vi "Main.vi"() -> ()   [LabVIEW 2014]
uses:
  <vilib>/vision/NI_Vision_Development_Module.lvlib
  <vilib>/vision/Measure.llb/Edge Polarity.ctl
  <vilib>/vision/Measure.llb/Edge Options.ctl
  <vilib>/vision/Measure.llb/Edge New.ctl
panel:
  out "Size factor":dbl
  in  "Tab Control":enum32{"MCF", "Kapilara"}(tab)
  in  "Nr punktu":i32
  in  "HIDE / SHOW":bool
  in  "Pole widzenia":dbl
  in  "Próg dopasowania okręgu":dbl=35.0
  in  "START":bool
  out "Mniejsza oś":dbl
  out "Większa oś":dbl
  out "Ekscentryczność":dbl
  out "Kołowość":dbl
  out "Przesunięcie [um]":dbl
  out "Parametry":string[][](table)
  in  "File path":path
  in  "START 2":bool
  in  "Pole widzenia":dbl
  in  "File path 2":path
  out "Średnica zewnętrzna [um]":i16
  out "Średnica wewnętrzna [um]":dbl format="%#_3g"
  in  "Options":T3={"Search  Direction"=1, "Edge Options"={"Edge Polarity"=2, "Kernel Size"=3, "Width"=3, "Minimum Edge Strength"=35.0, "Interpolation Type"=enum."Bilinear Fixed", "Data Processing Method"=enum."Average"}, "Show Search Area"=FALSE, "Show Search Lines"=FALSE, "Show Edges Found"=FALSE, "Show Result"=TRUE, "Search Area Color"=16711680, "Search Lines Color"=255, "Edge Locations Color"=16776960, "Result Color"=2162432, "Overlay Group Name"=""} {"Search  Direction" items=["Outside to Inside", "Inside to Outside"]; "Edge Options"."Edge Polarity" items=["All Edges", "Rising Edges", "Falling Edges"]; "Edge Options"."Minimum Edge Strength" format="%.2f"; "Edge Options"."Width" step=2; "Edge Options"."Kernel Size" step=2}
  in  "STOP":bool
  out "Array 3":cluster{"Edge Info":T4, "Boolean":bool}[](array[cluster]) {"Edge Info"."Distance (Real-World)" format="%.2f"; "Edge Info"."Location (Real-World)"."Y" format="%.2g"; "Edge Info"."Location (Real-World)"."X" format="%.2f"; "Edge Info"."Noise" format="%.2f"; "Edge Info"."Location (Pixel)"."Y" format="%.2g"; "Edge Info"."Location (Pixel)"."X" format="%.2f"; "Edge Info"."Strength" format="%.2f"; "Edge Info"."Distance (Pixel)" format="%.2f"}
  out "Displayed image":T5(plugin-control)
  out "Points array":cluster{"Edge Info":T4, "Boolean":bool}[](array[cluster]) {"Edge Info"."Distance (Real-World)" format="%.2f"; "Edge Info"."Location (Real-World)"."Y" format="%.2g"; "Edge Info"."Location (Real-World)"."X" format="%.2f"; "Edge Info"."Noise" format="%.2f"; "Edge Info"."Location (Pixel)"."Y" format="%.2g"; "Edge Info"."Location (Pixel)"."X" format="%.2f"; "Edge Info"."Strength" format="%.2f"; "Edge Info"."Distance (Pixel)" format="%.2f"}
  out "Original image":T5(plugin-control)
  # "Kliknięcie na zdjęciu spowoduje zaznaczenie \nnajbliższego punktu (widocznego lub ukrytego).\n\nNaciśnięcie przycisku POKAŻ / UKRYJ \nlub DOWOLNEGO PRZYCISKU NA KLAWIATURZE \nspowoduje pokazanie / ukrycie zaznaczonego punktu. \n\nDo obliczeń brane są tylko punkty widoczne na zdjęciu."
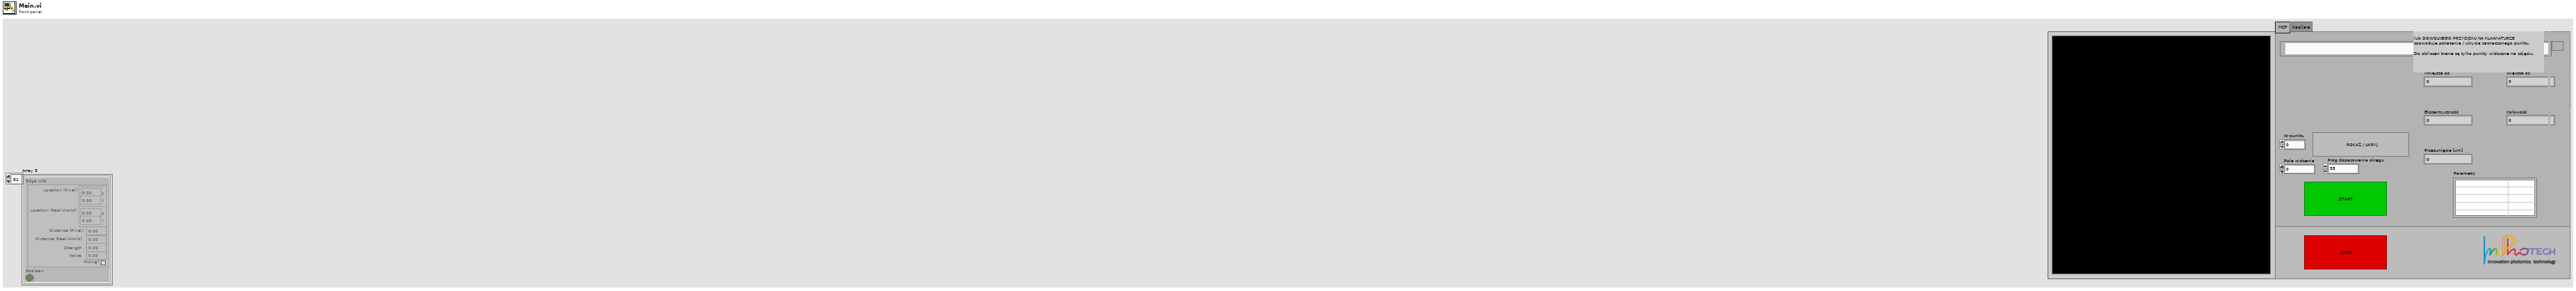
[diagram p1: front panel]
types:
  T1 = typedef "Edge Options.ctl" = cluster{"Edge Polarity":T2, "Kernel Size":u32, "Width":u32, "Minimum Edge Strength":sgl, "Interpolation Type":enum32{"Zero Order", "Bilinear", "Quadratic", "Cubic", "Bilinear Fixed"}, "Data Processing Method":enum32{"Average", "Median"}}
  T2 = typedef "Edge Polarity.ctl" = u32
  T3 = cluster{"Search  Direction":u32, "Edge Options":T1, "Show Search Area":bool, "Show Search Lines":bool, "Show Edges Found":bool, "Show Result":bool, "Search Area Color":u32, "Search Lines Color":u32, "Edge Locations Color":u32, "Result Color":u32, "Overlay Group Name":string}
  T4 = typedef "Edge New.ctl" = cluster{"Location (Pixel)":cluster{"X":sgl, "Y":sgl}, "Location (Real-World)":cluster{"X":sgl, "Y":sgl}, "Distance (Pixel)":dbl, "Distance (Real-World)":dbl, "Strength":dbl, "Noise":dbl, "Rising?":bool}
  T5 = typedef "IMAQ Image.ctl" = refnum<image>
  T6 = typedef "IMAQ Circle" = cluster{"Center X":i32, "Center Y":i32, "Inner Radius":i32, "Outer Radius":i32, "Start Angle":dbl, "End Angle":dbl}
  T7 = cluster{dbl, dbl, dbl, dbl, "Start Angle":dbl, "End Angle":dbl}
  T8 = typedef "ROI Descriptor" = cluster{"Global Rectangle":i32[], "Contours":cluster{"ID":enum32{"External", "Internal"}, "Type":u32, "Coordinates":i32[]}[]}
  T9 = cluster{"Center (Pixels)":cluster{"X":sgl, "Y":sgl}, "Radius (Pixels)":dbl, "Center (Real-World)":cluster{"X":sgl, "Y":sgl}, "Radius (Real-World)":dbl, "Roundness (Real-World)":dbl, "Average Strength":dbl, "Average SNR (dB)":dbl}
  T10 = cluster{"Center":cluster{"X":sgl, "Y":sgl}, "Major Axis":cluster{"Point 1":cluster{"X":sgl, "Y":sgl}, "Point 2":cluster{"X":sgl, "Y":sgl}}, "Minor Axis":cluster{"Point 1":cluster{"X":sgl, "Y":sgl}, "Point 2":cluster{"X":sgl, "Y":sgl}}}
  T11 = enum32{"Zero Order", "Bilinear", "Quadratic", "Cubic", "Bilinear Fixed"}
  T12 = cluster{"Edge Polarity":T2, "Kernel Size":u32, "Width":u32, "NewVal":dbl, "Interpolation Type":enum32{"Zero Order", "Bilinear", "Quadratic", "Cubic", "Bilinear Fixed"}, "Data Processing Method":enum32{"Average", "Median"}}
  T13 = cluster{"Search  Direction":u32, cluster{"Edge Polarity":T2, "Kernel Size":u32, "Width":u32, "NewVal":dbl, "Interpolation Type":enum32{"Zero Order", "Bilinear", "Quadratic", "Cubic", "Bilinear Fixed"}, "Data Processing Method":enum32{"Average", "Median"}}, "Show Search Area":bool, "Show Search Lines":bool, "Show Edges Found":bool, "Show Result":bool, "Search Area Color":u32, "Search Lines Color":u32, "Edge Locations Color":u32, "Result Color":u32, "Overlay Group Name":string}
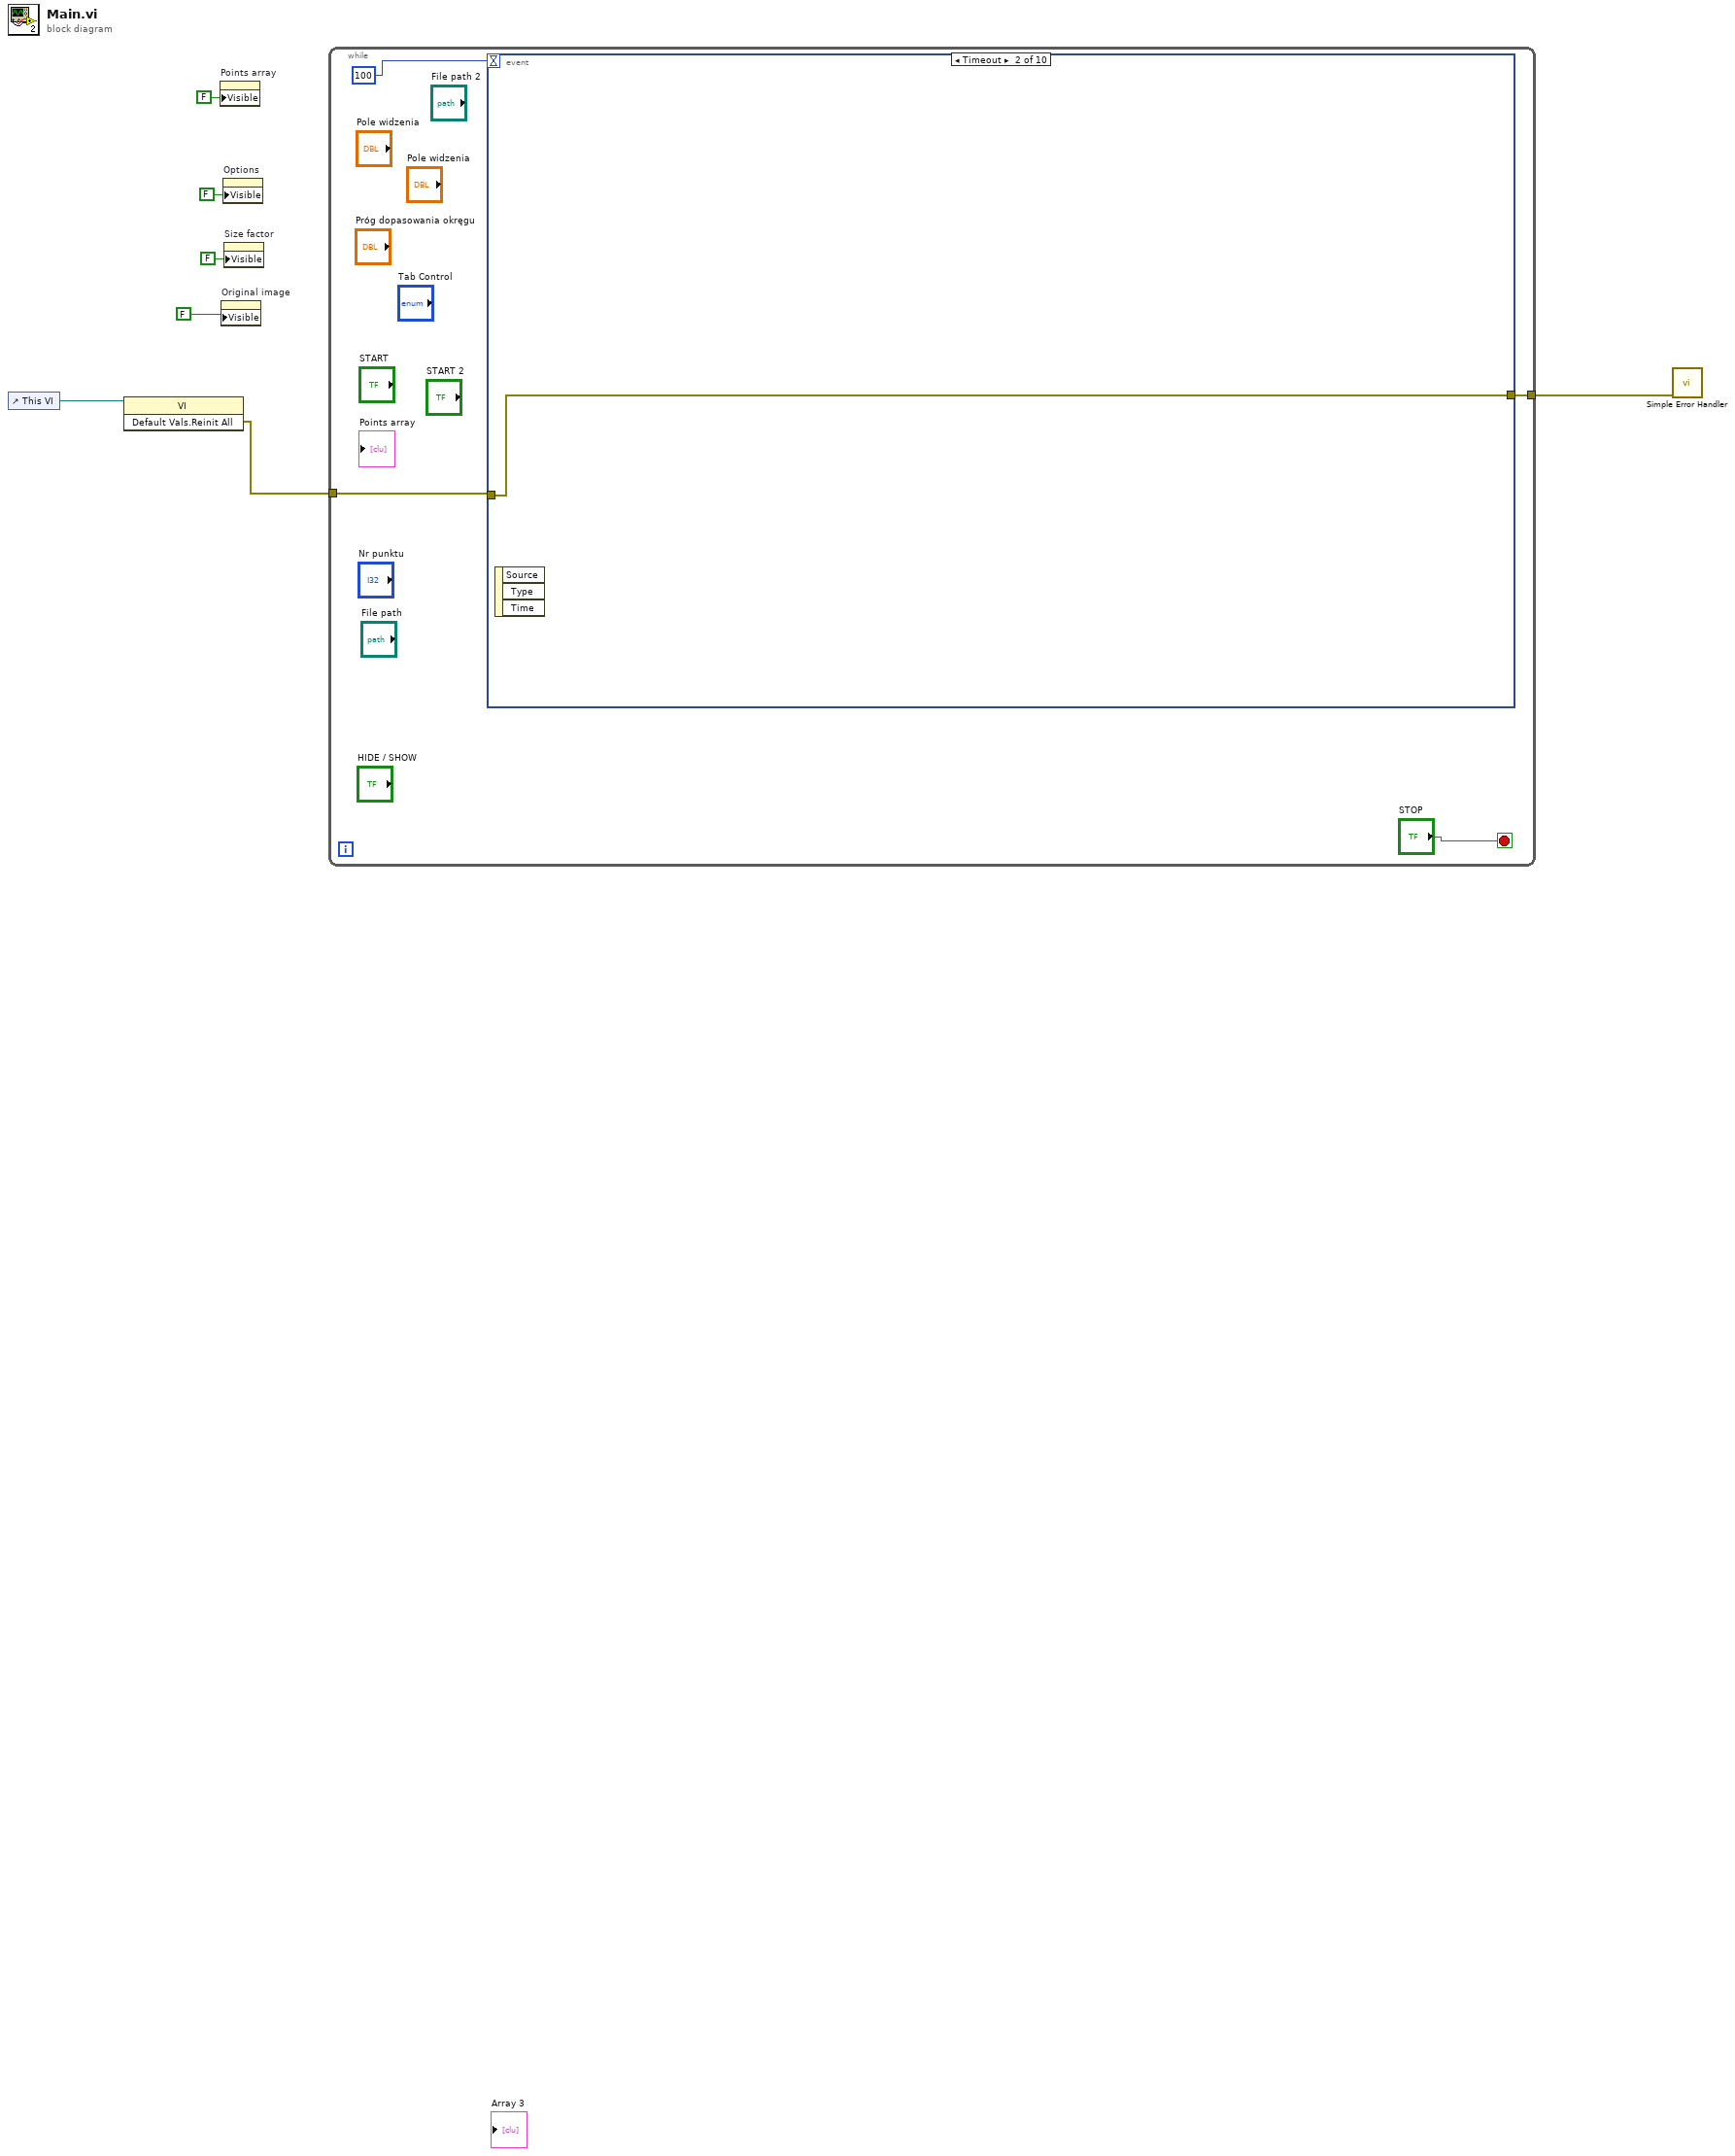
[diagram p0: block diagram]
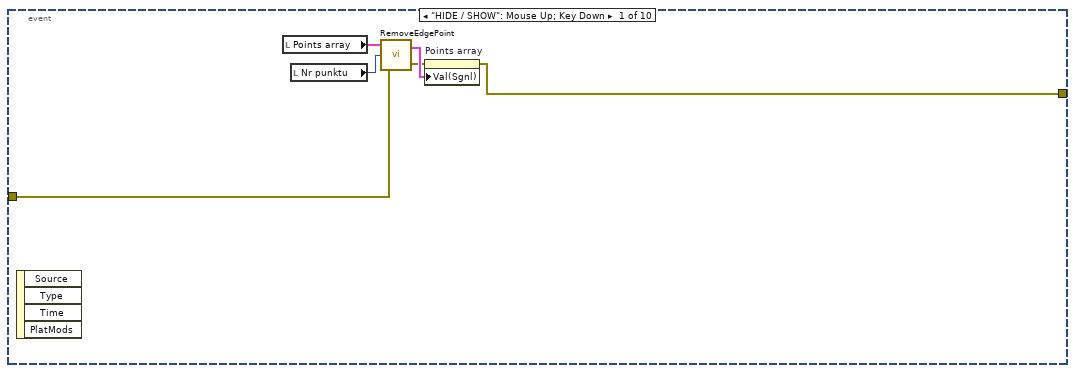
[diagram p2: hidden frame]
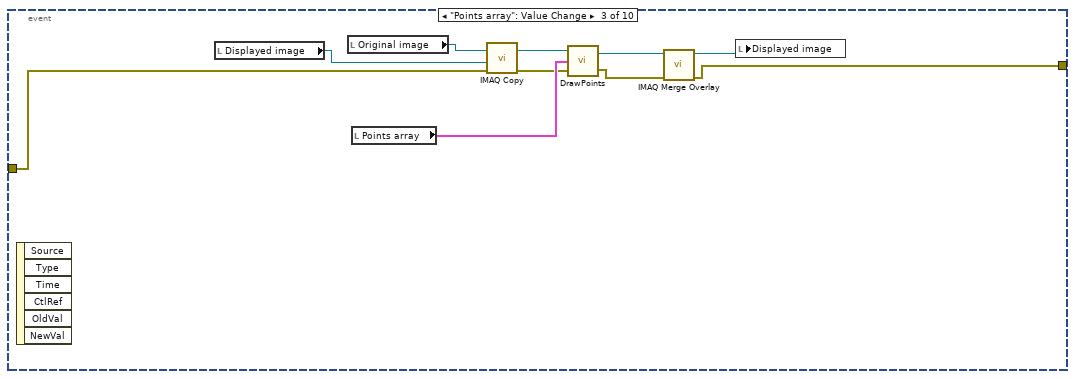
[diagram p3: hidden frame]
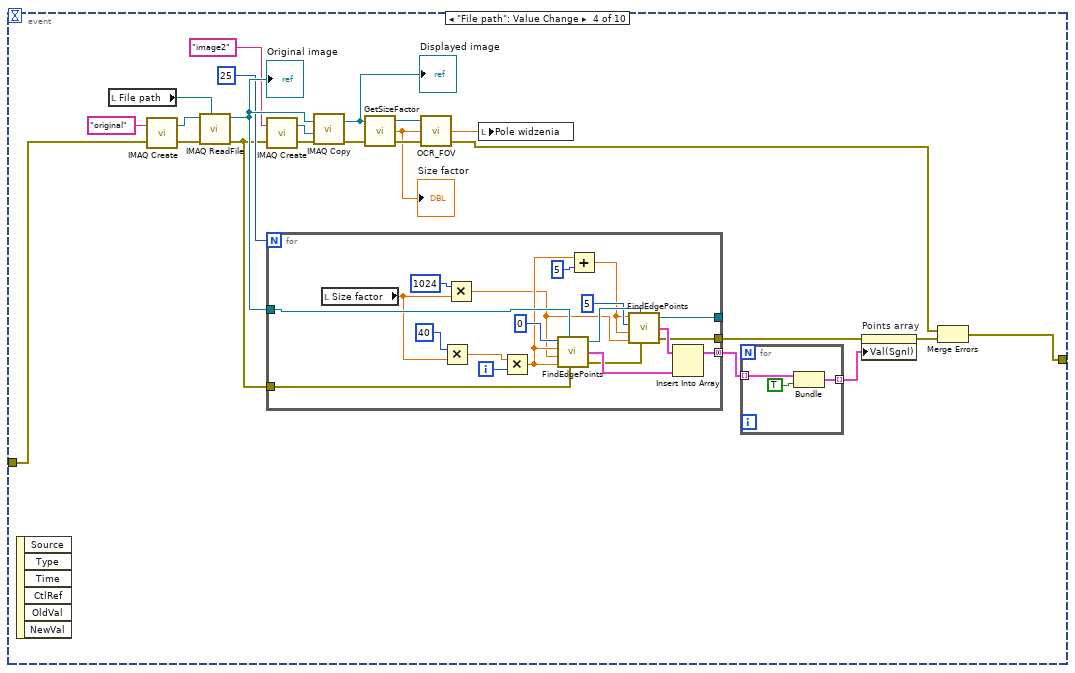
[diagram p4: hidden frame]
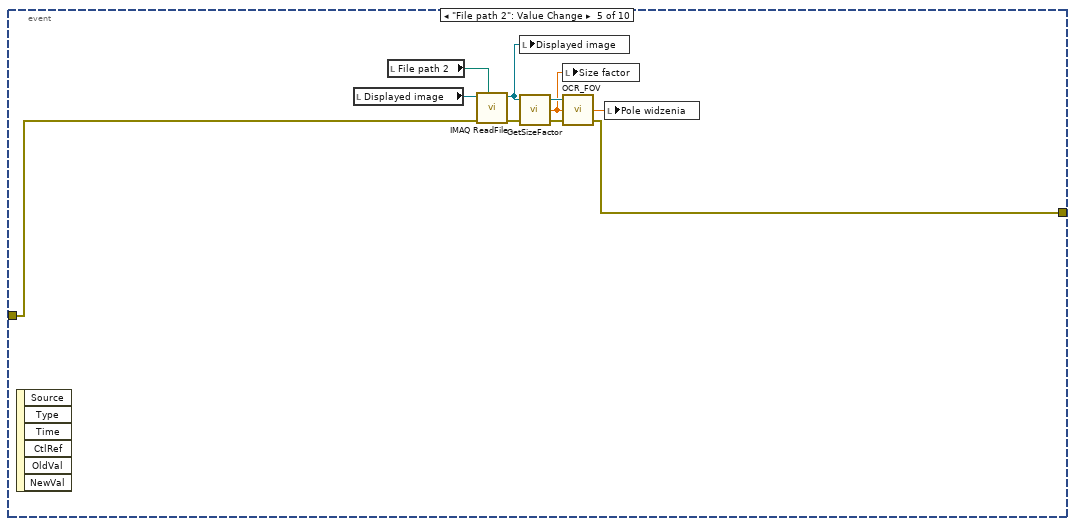
[diagram p5: hidden frame]
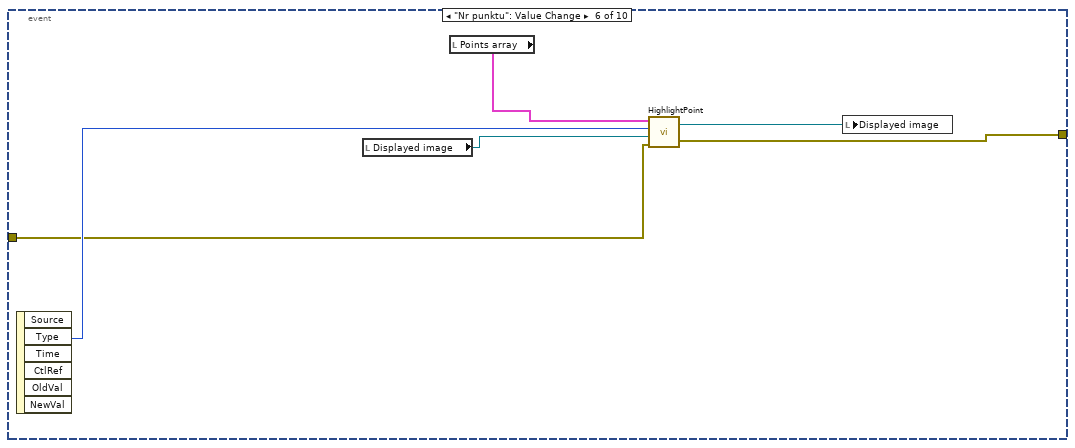
[diagram p6: hidden frame]
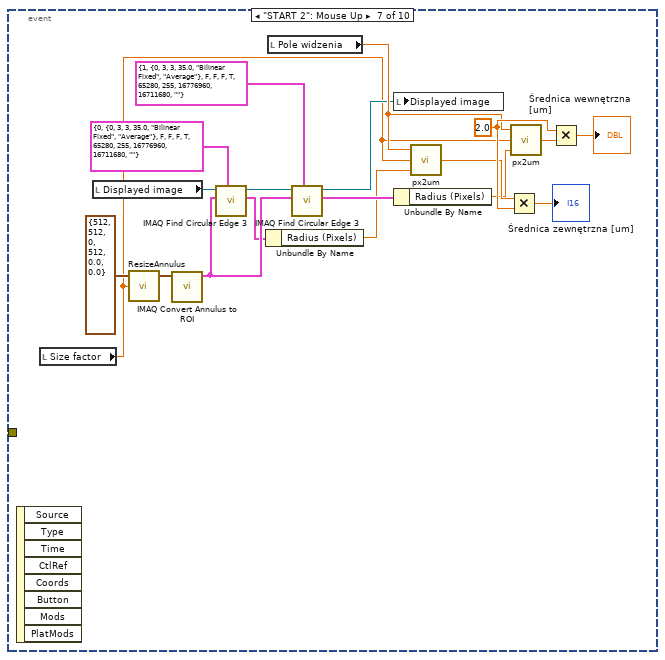
[diagram p7: hidden frame]
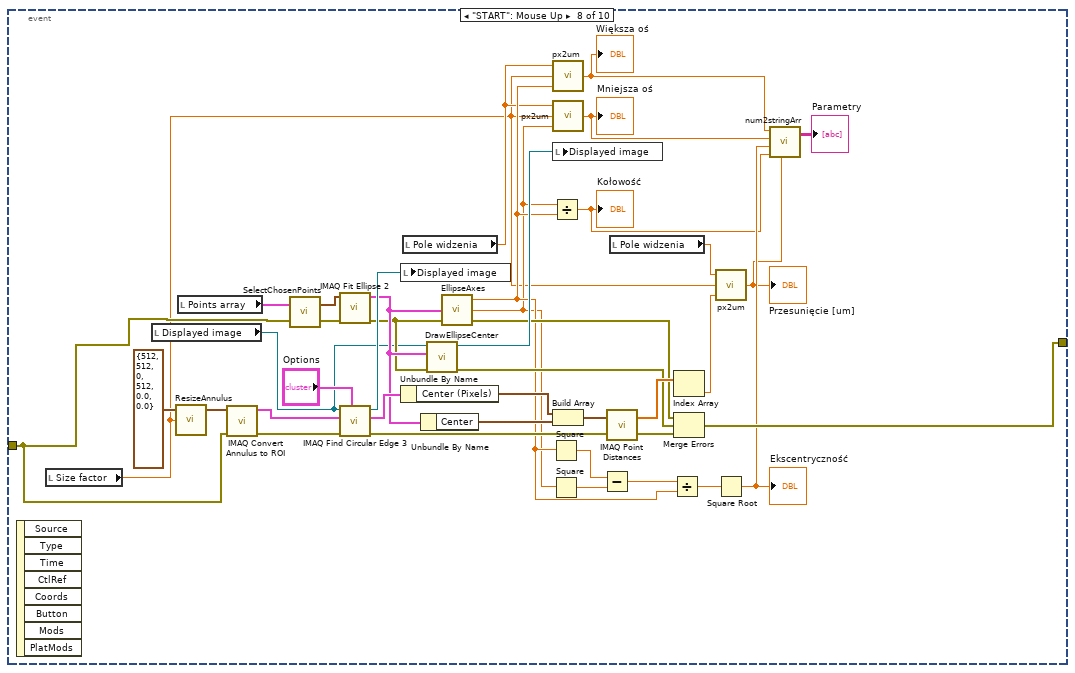
[diagram p8: hidden frame]
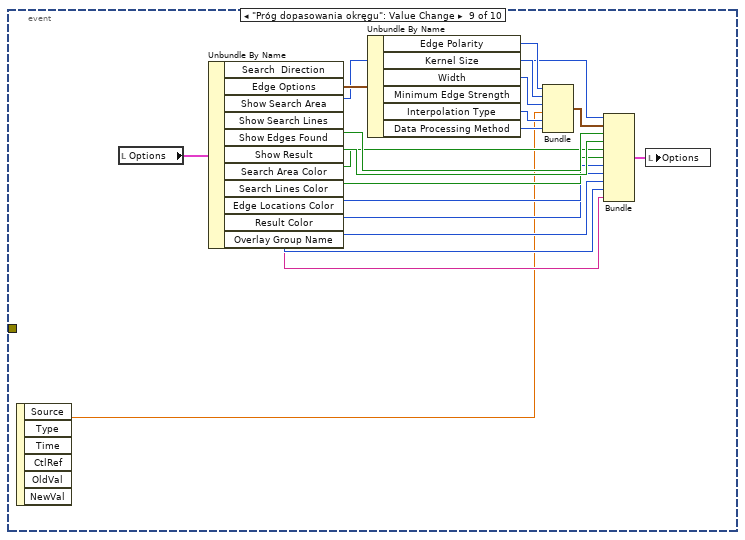
[diagram p9: hidden frame]
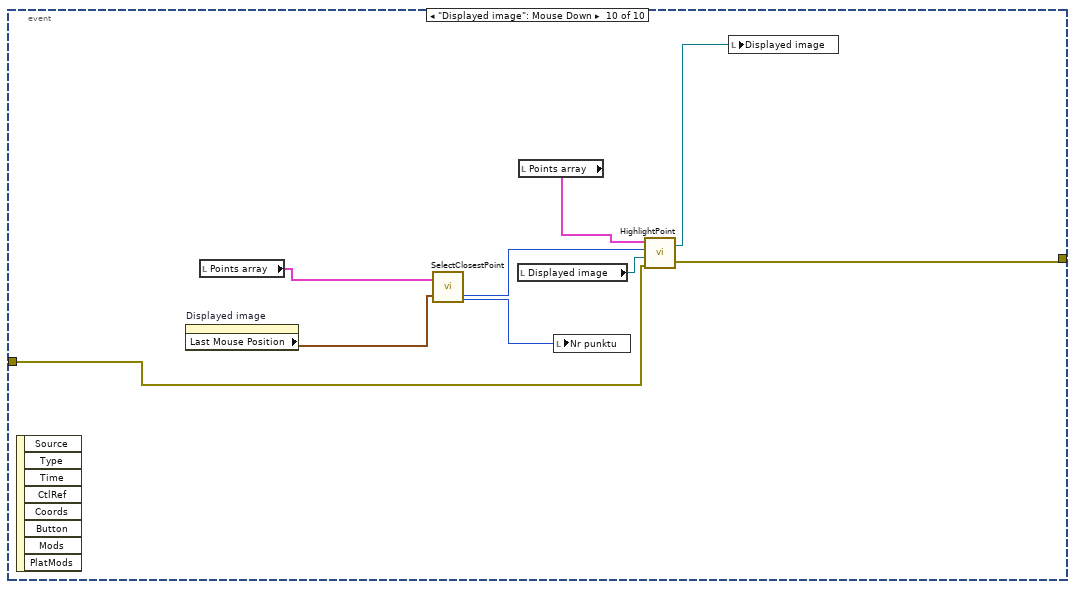
[diagram p10: hidden frame]
diagram:
  n1 = control-ref of="This VI"() -> (w5:refnum<vi>)
  n2 = invoke class="VI" method="Default Vals.Reinit All"(reference=w5) -> (error out=w4:errorcluster)  [unwired: 2 in, 2 out]
  n3 = property on="Points array" class="Arr (strict)"("Visible"=FALSE) -> ()  [unwired: 2 in, 2 out]
  n4 = property on="Original image" class="ImageControl"("Visible"=FALSE) -> ()  [unwired: 2 in, 2 out]
  n5 = property on="Options" class="Clust (strict)"("Visible"=FALSE) -> ()  [unwired: 2 in, 2 out]
  n6 = property on="Size factor" class="DigNum (strict)"("Visible"=FALSE) -> ()  [unwired: 2 in, 2 out]
  n7 = while {
    tunnel: w4 -> [w9]
    tunnel: [w8] -> w3
    stop <- "STOP" stop-if-true
    n8 = event shown="[1] Timeout" {
      selector: _ -> [_ _ _ _ _ _ _ _ _ _]
      dyn-events: _ -> [_ _ _ _ _ _ _ _ _ _]
      timeout: 100 -> [_ _ _ _ _ _ _ _ _ _]
      tunnel: w9 -> [w12 w18 w22 w42 w82 w86 _ w130 _ w170]
      tunnel: [w13 w18 w19 w38 w81 w85 _ w123 _ w171] -> w8
      event "HIDE / SHOW": Mouse Up; Key Down {
        n9 = event-data() -> ()  [unwired: 1 in, 4 out]
        n10 = local read "Points array"() -> (w17:cluster{"Edge Info":T4, "Boolean":bool}[])
        n11 = local read "Nr punktu"() -> (w16:i32)
        n12 = call "RemoveEdgePoint.vi"("error constant"=w12, "index"=w16, "array"=w17) -> ("error constant 2"=w14:errorcluster, "output array"=w15:cluster{"Edge Info":T4, "Boolean":bool}[])
        n13 = property on="Points array" class="Arr (strict)"(error in=w14, "Val(Sgnl)"=w15) -> (error out=w13:errorcluster)  [unwired: 1 in, 1 out]
      }
      event Timeout {
        n14 = event-data() -> ()  [unwired: 1 in, 3 out]
      }
      event "Points array": Value Change {
        n15 = event-data() -> ()  [unwired: 1 in, 6 out]
        n16 = local read "Displayed image"() -> (w27:T5)
        n17 = local read "Original image"() -> (w26:T5)
        n18 = local read "Points array"() -> (w23:cluster{"Edge Info":T4, "Boolean":bool}[])
        n19 = call "IMAQ Copy"("error in (no error)"=w22, "Image Dst"=w27, "Image Src"=w26) -> ("error out"=w21:errorcluster, "Image Dst Out"=w28:T5)  [unwired: 3 in]
        n20 = call "DrawPoints.vi"("error in (no error)"=w21, "Points"=w23, "Image in"=w28) -> ("error out"=w20:errorcluster, "Image Out"=w24:T5)
        n21 = call "IMAQ Merge Overlay"("error in (no error)"=w20, "Image Src"=w24) -> ("error out"=w19:errorcluster, "Image Dst Out"=w25:T5)  [unwired: 8 in]
        n22 = local write "Displayed image"(w25) -> ()
      }
      event "File path": Value Change {
        n23 = event-data() -> ()  [unwired: 1 in, 6 out]
        n24 = local read "File path"() -> (w44:path)
        n25 = call "IMAQ Create"("Image Name"="original", "error in (no error)"=w42) -> ("New Image"=w48:T5, "error out"=w41:errorcluster)  [unwired: 3 in]
        n26 = call "IMAQ ReadFile"("File Path"=w44, "error in (no error)"=w41, "Image"=w48) -> ("error out"=w37:errorcluster, "Image Out"=w51:T5)  [unwired: 4 in, 3 out]
        "Original image" <- w51
        n27 = call "IMAQ Create"("Image Name"="image2", "error in (no error)"=w37) -> ("New Image"=w50:T5, "error out"=w40:errorcluster)  [unwired: 3 in]
        n28 = for {
          N: 25 -> [_]
          tunnel: [w74] -> w45 mode=concatenating
          tunnel: [w69] -> _
          tunnel: w51 -> [w66]
          tunnel: w37 -> [w61]
          tunnel: [w60] -> w36
          i -> [w67]
          n29 = local read "Size factor"() -> (w55:dbl)
          n30 = Multiply(x=40, y=w55) -> (x*y=w57:dbl)
          n31 = Multiply(x=1024, y=w55) -> (x*y=w58:dbl)
          n32 = Multiply(x=w57, y=w67) -> (x*y=w64:dbl)
          n33 = call "FindEdgePoints.vi"("X1"=0, "Image in"=w66, "Y1"=w64, "X2"=w58, "error in (no error)"=w61, "Y2"=w64) -> ("Image out"=w73:T5, "Edge point"=w71:T4[], "error out"=w70:errorcluster)
          n34 = Add(x=w64, y=5) -> (x+y=w62:dbl)
          n35 = call "FindEdgePoints.vi"("X1"=w62, "Image in"=w73, "Y1"=5, "X2"=w62, "error in (no error)"=w70, "Y2"=w58) -> ("Image out"=w69:T5, "Edge point"=w72:T4[], "error out"=w60:errorcluster)
          n36 = Insert Into Array(array=w72, new element=w71) -> (w74:T4[])  [unwired: 1 in]
        }
        n37 = call "IMAQ Copy"("error in (no error)"=w40, "Image Dst"=w50, "Image Src"=w51) -> ("error out"=w33:errorcluster, "Image Dst Out"=w32:T5)  [unwired: 3 in]
        "Displayed image" <- w32
        n38 = call "GetSizeFactor.vi"("error in (no error)"=w33, "IMAQImage"=w32) -> ("error out"=w30:errorcluster, "Size factor"=w29:dbl, "IMAQImage 2"=w31:T5)  [unwired: 1 in]
        "Size factor" <- w29
        n39 = call "OCR_FOV.vi"("error in"=w30, "Size factor"=w29, "Image in"=w31) -> ("error out"=w35:errorcluster, "FOV"=w34:dbl)  [unwired: 1 out]
        n40 = local write "Pole widzenia"(w34) -> ()
        n41 = for {
          tunnel: w45 -> [w54] mode=indexing
          tunnel: [w53] -> w43 mode=indexing
          n42 = Bundle("Edge Info"=w54, TRUE) -> (w53:cluster{"Edge Info":T4, bool})  [unwired: 1 in]
        }
        n43 = property on="Points array" class="Arr (strict)"(error in=w36, "Val(Sgnl)"=w43) -> (error out=w39:errorcluster)  [unwired: 1 in, 1 out]
        n44 = Merge Errors(w35, w39) -> (w38:errorcluster)
      }
      event "File path 2": Value Change {
        n45 = event-data() -> ()  [unwired: 1 in, 6 out]
        n46 = local read "Displayed image"() -> (w83:T5)
        n47 = local read "File path 2"() -> (w84:path)
        n48 = call "IMAQ ReadFile"("File Path"=w84, "error in (no error)"=w82, "Image"=w83) -> ("error out"=w78:errorcluster, "Image Out"=w79:T5)  [unwired: 4 in, 3 out]
        n49 = local write "Displayed image"(w79) -> ()
        n50 = call "GetSizeFactor.vi"("error in (no error)"=w78, "IMAQImage"=w79) -> ("error out"=w76:errorcluster, "Size factor"=w75:dbl, "IMAQImage 2"=w77:T5)  [unwired: 1 in]
        n51 = local write "Size factor"(w75) -> ()
        n52 = call "OCR_FOV.vi"("error in"=w76, "Size factor"=w75, "Image in"=w77) -> ("error out"=w81:errorcluster, "FOV"=w80:dbl)  [unwired: 1 out]
        n53 = local write "Pole widzenia"(w80) -> ()
      }
      event "Nr punktu": Value Change {
        n54 = event-data() -> ("NewVal"=w89:i32)  [unwired: 1 in, 5 out]
        n55 = local read "Displayed image"() -> (w88:T5)
        n56 = local read "Points array"() -> (w90:cluster{"Edge Info":T4, "Boolean":bool}[])
        n57 = call "HighlightPoint.vi"("error in"=w86, "Image In"=w88, "index"=w89, "points"=w90) -> ("error out"=w85:errorcluster, "Image Out"=w87:T5)
        n58 = local write "Displayed image"(w87) -> ()
      }
      event "START 2": Mouse Up {
        w109 = 2.0 ("x")
        n59 = event-data() -> ()  [unwired: 1 in, 8 out]
        n60 = local read "Size factor"() -> (w91:dbl)
        n61 = local read "Displayed image"() -> (w104:T5)
        n62 = call "ResizeAnnulus.vi"("y"=w91, "Input Annulus"=T6 {"Center X"=512, "Center Y"=512, "Inner Radius"=0, "Outer Radius"=512, "Start Angle"=0.0, "End Angle"=0.0} ("Annulus")) -> ("Output Annulus"=w93:T7)  [unwired: 3 in]
        n63 = call "IMAQ Convert Annulus to ROI"("Annulus"=w93) -> ("ROI Descriptor"=w102:T8)  [unwired: 8 in, 1 out]
        n64 = call "IMAQ Find Circular Edge 3"("Options"=T3 {"Search  Direction"=0, "Edge Options"={"Edge Polarity"=0, "Kernel Size"=3, "Width"=3, "Minimum Edge Strength"=35.0, "Interpolation Type"=enum."Bilinear Fixed", "Data Processing Method"=enum."Average"}, "Show Search Area"=FALSE, "Show Search Lines"=FALSE, "Show Edges Found"=FALSE, "Show Result"=TRUE, "Search Area Color"=65280, "Search Lines Color"=255, "Edge Locations Color"=16776960, "Result Color"=16711680, "Overlay Group Name"=""}, "ROI Descriptor"=w102, "Image"=w104) -> ("Fitted Circle"=w98:T9, "Image Out"=w99:T5)  [unwired: 4 in, 3 out]
        n65 = Unbundle By Name(w98) -> ("Radius (Pixels)"=w96:dbl)
        n66 = local read "Pole widzenia"() -> (w103:dbl)
        n67 = call "IMAQ Find Circular Edge 3"("Options"=T3 {"Search  Direction"=1, "Edge Options"={"Edge Polarity"=0, "Kernel Size"=3, "Width"=3, "Minimum Edge Strength"=35.0, "Interpolation Type"=enum."Bilinear Fixed", "Data Processing Method"=enum."Average"}, "Show Search Area"=FALSE, "Show Search Lines"=FALSE, "Show Edges Found"=FALSE, "Show Result"=TRUE, "Search Area Color"=65280, "Search Lines Color"=255, "Edge Locations Color"=16776960, "Result Color"=16711680, "Overlay Group Name"=""}, "ROI Descriptor"=w102, "Image"=w99) -> ("Fitted Circle"=w97:T9, "Image Out"=w94:T5)  [unwired: 4 in, 3 out]
        n68 = local write "Displayed image"(w94) -> ()
        n69 = Unbundle By Name(w97) -> ("Radius (Pixels)"=w95:dbl)
        n70 = call "px2um.vi"("px"=w96, "Size factor"=w91, "Field of view"=w103) -> ("um"=w105:dbl)
        n71 = Multiply(x=w105, y=w109) -> (x*y=→"Średnica zewnętrzna [um]":dbl)
        n72 = call "px2um.vi"("px"=w95, "Size factor"=w91, "Field of view"=w103) -> ("um"=w107:dbl)
        n73 = Multiply(x=w109, y=w107) -> (x*y=→"Średnica wewnętrzna [um]":dbl)
      }
      event "START": Mouse Up {
        n74 = event-data() -> ()  [unwired: 1 in, 8 out]
        n75 = local read "Size factor"() -> (w110:dbl)
        n76 = local read "Displayed image"() -> (w122:T5)
        n77 = call "ResizeAnnulus.vi"("y"=w110, "Input Annulus"=T6 {"Center X"=512, "Center Y"=512, "Inner Radius"=0, "Outer Radius"=512, "Start Angle"=0.0, "End Angle"=0.0} ("Annulus")) -> ("Output Annulus"=w111:T7)  [unwired: 3 in]
        n78 = local read "Points array"() -> (w148:cluster{"Edge Info":T4, "Boolean":bool}[])
        n79 = call "IMAQ Convert Annulus to ROI"("error in (no error)"=w130, "Annulus"=w111) -> ("error out"=w129:errorcluster, "ROI Descriptor"=w145:T8)  [unwired: 7 in]
        n80 = call "SelectChosenPoints.vi"("error in (no error)"=w130, "Points array"=w148) -> ("error out"=w131:errorcluster, "array"=w147:cluster{"X":sgl, "Y":sgl}[])
        n81 = call "IMAQ Fit Ellipse 2"("error in (no error)"=w131, "Radial Points"=w147) -> ("error out"=w127:errorcluster, "Ellipse"=w142:T10)  [unwired: 4 in, 4 out]
        n82 = call "IMAQ Find Circular Edge 3"("Options"="Options", "error in (no error)"=w129, "ROI Descriptor"=w145, "Image"=w122) -> ("error out"=w128:errorcluster, "Fitted Circle"=w143:T9, "Image Out"=w144:T5)  [unwired: 3 in, 2 out]
        n83 = local write "Displayed image"(w144) -> ()
        n84 = Unbundle By Name(w143) -> ("Center (Pixels)"=w141:cluster{"X":sgl, "Y":sgl})
        n85 = local read "Pole widzenia"() -> (w120:dbl)
        n86 = Unbundle By Name(w142) -> ("Center"=w140:cluster{"X":sgl, "Y":sgl})
        n87 = call "DrawEllipseCenter.vi"("error in"=w127, "Ellipse"=w142, "Image in"=w122) -> ("error out"=w126:errorcluster, "Image out"=w149:T5)  [unwired: 7 in]
        n88 = call "EllipseAxes.vi"("error in (no error)"=w127, "input cluster"=w142) -> ("error out"=w124:errorcluster, "Minor axis"=w119:dbl, "Major axis"=w121:dbl)  [unwired: 1 in]
        n89 = Square(x=w121) -> (x^2=w135:dbl)
        n90 = Square(x=w119) -> (x^2=w134:dbl)
        n91 = Divide(x=w119, y=w121) -> (x/y=w114:dbl)
        "Kołowość" <- w114
        n92 = call "px2um.vi"("px"=w121, "Size factor"=w110, "Field of view"=w120) -> ("um"=w117:dbl)
        "Większa oś" <- w117
        n93 = call "px2um.vi"("px"=w119, "Size factor"=w110, "Field of view"=w120) -> ("um"=w116:dbl)
        "Mniejsza oś" <- w116
        n94 = local write "Displayed image"(w149) -> ()
        n95 = Build Array(w141, w140) -> (w138:cluster{"X":sgl, "Y":sgl}[])
        n96 = Subtract(x=w135, y=w134) -> (x-y=w133:dbl)
        n97 = call "IMAQ Point Distances"("Points"=w138, "error in (no error)"=w128) -> ("Distances"=w137:sgl[], "error out"=w125:errorcluster)  [unwired: 3 in]
        n98 = local read "Pole widzenia"() -> (w139:dbl)
        n99 = Divide(x=w133, y=w121) -> (x/y=w132:dbl)
        n100 = Index Array(array=w137) -> (element=w136:sgl)  [unwired: 1 in]
        n101 = Merge Errors(w124, w126, w125) -> (w123:errorcluster)
        n102 = call "px2um.vi"("px"=w136, "Size factor"=w110, "Field of view"=w139) -> ("um"=w113:dbl)
        "Przesunięcie [um]" <- w113
        n103 = Square Root(x=w132) -> (sqrt(x)=w115:dbl)
        "Ekscentryczność" <- w115
        n104 = call "num2stringArr.vi"("item 1"=w117, "item 2"=w116, "item 3"=w115, "item 4"=w114, "item5"=w113) -> ("Array"=→"Parametry":string[][])  [unwired: 1 in]
      }
      event "Próg dopasowania okręgu": Value Change {
        n105 = event-data() -> ("NewVal"=w150:dbl)  [unwired: 1 in, 5 out]
        n106 = local read "Options"() -> (w169:T3)
        n107 = Unbundle By Name(w169) -> ("Search  Direction"=w162:u32, "Edge Options"=w168:T1, "Show Search Area"=w160:bool, "Show Search Lines"=w159:bool, "Show Edges Found"=w158:bool, "Show Result"=w157:bool, "Search Area Color"=w156:u32, "Search Lines Color"=w155:u32, "Edge Locations Color"=w154:u32, "Result Color"=w153:u32, "Overlay Group Name"=w152:string)
        n108 = Unbundle By Name(w168) -> ("Edge Polarity"=w167:T2, "Kernel Size"=w166:u32, "Width"=w165:u32, "Interpolation Type"=w164:T11, "Data Processing Method"=w163:enum32{"Average", "Median"})  [unwired: 1 out]
        n109 = Bundle("Edge Polarity"=w167, "Kernel Size"=w166, "Width"=w165, "NewVal"=w150, "Interpolation Type"=w164, "Data Processing Method"=w163) -> (w161:T12)  [unwired: 1 in]
        n110 = Bundle("Search  Direction"=w162, w161, "Show Search Area"=w160, "Show Search Lines"=w159, "Show Edges Found"=w158, "Show Result"=w157, "Search Area Color"=w156, "Search Lines Color"=w155, "Edge Locations Color"=w154, "Result Color"=w153, "Overlay Group Name"=w152) -> (w151:T13)  [unwired: 1 in]
        n111 = local write "Options"(w151) -> ()
      }
      event "Displayed image": Mouse Down {
        n112 = event-data() -> ()  [unwired: 1 in, 8 out]
        n113 = property on="Displayed image" class="ImageControl"() -> ("Last Mouse Position"=w174:cluster{"X":i32, "Y":i32})  [unwired: 2 in, 2 out]
        n114 = local read "Points array"() -> (w173:cluster{"Edge Info":T4, "Boolean":bool}[])
        n115 = call "SelectClosestPoint.vi"("Mouse Position"=w174, "Points"=w173) -> ("Point index"=w172:i32)
        n116 = local read "Displayed image"() -> (w175:T5)
        n117 = local read "Points array"() -> (w177:cluster{"Edge Info":T4, "Boolean":bool}[])
        n118 = local write "Nr punktu"(w172) -> ()
        n119 = call "HighlightPoint.vi"("error in"=w170, "Image In"=w175, "index"=w172, "points"=w177) -> ("error out"=w171:errorcluster, "Image Out"=w176:T5)
        n120 = local write "Displayed image"(w176) -> ()
      }
    }
  }
  n121 = call <vilib>:"Simple Error Handler.vi"("error in (no error)"=w3) -> ()  [unwired: 4 in, 5 out]
